vi "4461 Autophase.vi"(8 "error in (no error)":errorcluster, 9 "Boolean":bool, 10 "Results":T1 {"Results (Dictionary)"."value" format="%#_6p"}, 11 "Instrument.DAQ in":refnum<class "Instrument.DAQ.lvclass">) -> (0 "error out":errorcluster, 3 "Instrument.DAQ out":refnum<class "Instrument.DAQ.lvclass">)   [LabVIEW 2019, in "Instrument.DAQ.lvclass"]
uses:
  Instrument.DAQ.lvclass
  Typedefs/Results--Cluster.ctl
  Instrument.Lockin/Typedefs/Results Type--Enum.ctl
  Instrument.DAQ.lvclass/Instrument.DAQ.ctl
  <vilib>/addons/control/pid/pid.llb/PID (DBL Array).vi
  Instrument.Lockin/Instrument.Lockin.lvclass
  <vilib>/addons/control/pid/NI_PID_pid.lvlib
  <vilib>/addons/control/pid/pid.llb/PID Control Input Filter (DBL).vi
panel:
  out "output":dbl[](array[numeric]) format="%.2f"
  in  "D":dbl=0.019999999999999997 format="%.3f"
  in  "I":dbl=0.6 format="%.3f"
  in  "P":dbl=0.5 format="%.2f"
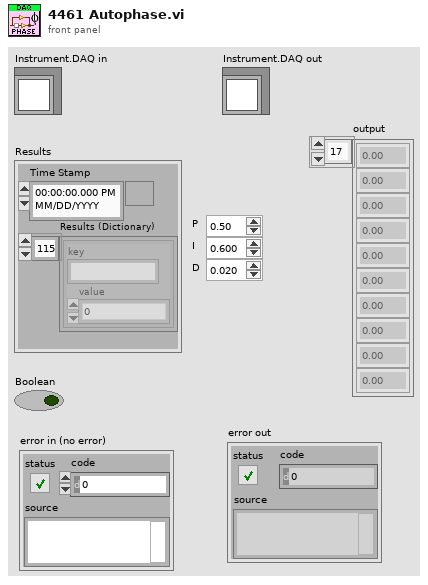
[diagram p1: front panel]
types:
  T1 = typedef "Instrument.DAQ.lvclass/Results--Cluster.ctl" = cluster{"Time Stamp":timestamp, "Results (Dictionary)":cluster{"key":string, "value":dbl}[]}
  T2 = cluster{"proportional gain (Kc)":dbl, "integral time (Ti, min)":dbl, "derivative time (Td, min)":dbl}
  T3 = typedef "Instrument.Lockin.lvclass/Results Type--Enum.ctl" = enum16{"X", "Y", "R", "Theta", "Mean"}
  T4 = typedef "Instrument.DAQ.lvclass/AO.Channel--Cluster--Array.ctl" = T5[]
  T5 = typedef "Instrument.DAQ.lvclass/AO.Channel--Cluster.ctl" = cluster{"Enable?":bool, "Channel":i32, "Amplitude":dbl, "Offset":dbl, "Frequency":dbl, "Phase":dbl, "Function":T6, "Sweeping?":bool}
  T6 = typedef "Instrument.DAQ.lvclass/AO.Channel.Function--Enum.ctl" = enum16{"Sine", "Triangle", "Square"}
  T7 = cluster{"proportional gain (Kc)":dbl, "integral time (Ti, min)":dbl, "derivative time (Td, min)":dbl}[]
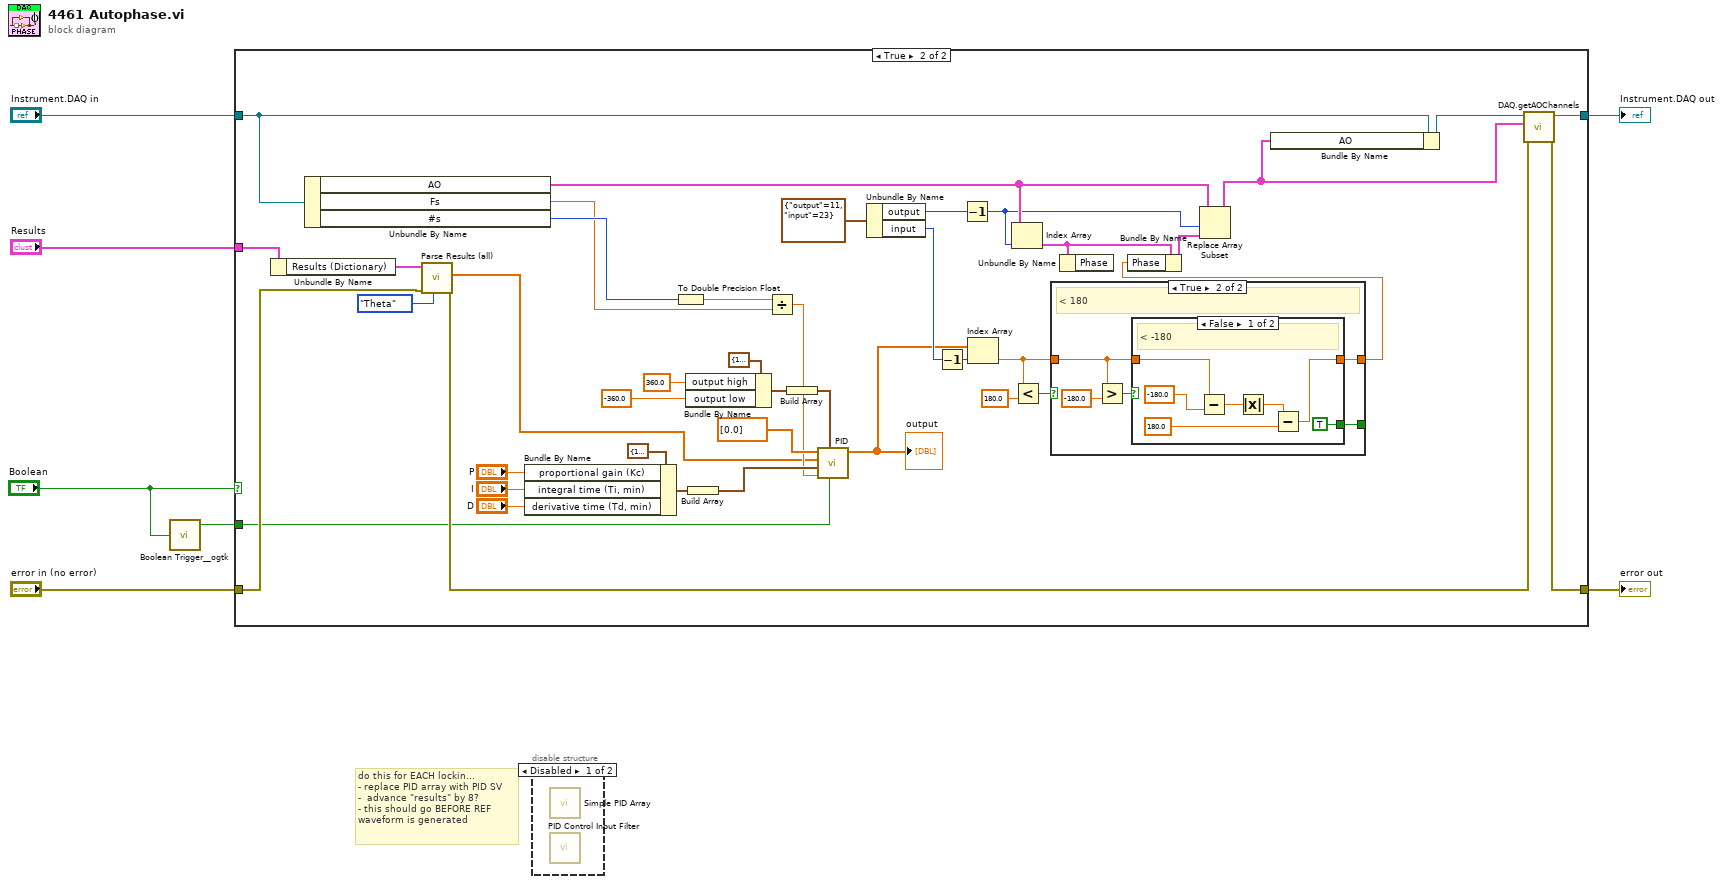
[diagram p0: block diagram]
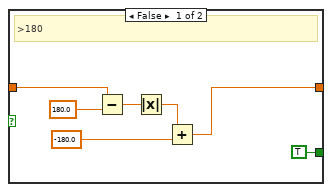
[diagram p3: hidden frame]
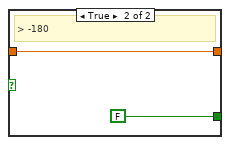
[diagram p4: hidden frame]
diagram:
  # "do this for EACH lockin...\n- replace PID array with PID SV\n-  advance \"results\" by 8?\n- this should go BEFORE REF\nwaveform is generated"
  n1 = call <userlib>:"Boolean Trigger__ogtk.vi"("Boolean Input"="Boolean") -> ("Rising Edge"=w1:bool)  [unwired: 1 in, 1 out]
  n2 = case shown="True" "Boolean" {
    tunnel: "Instrument.DAQ in" -> [w9 w50]
    tunnel: "Results" -> [_ w49]
    tunnel: "error in (no error)" -> [w8 w48]
    tunnel: [w9 w47] -> w4
    tunnel: [w8 w11] -> w3
    tunnel: w1 -> [_ w10]
    frame False {
    }
    frame True {
      n3 = Unbundle By Name(w49) -> ("Results (Dictionary)"=w46:cluster{"key":string, "value":dbl}[])
      n4 = Unbundle By Name(w50) -> ("AO"=w30:T4, "Fs"=w20:dbl, "#s"=w21:i32)
      n5 = call "Parse Results (all).vi"("Type"=Results_Type--Enum."Theta", "error in (no error)"=w48, "Results (Dictionary)"=w46) -> ("error out"=w43:errorcluster, "Data"=w12:dbl[])  [unwired: 5 in, 2 out]
      n6 = Bundle By Name(cluster=T2 {"proportional gain (Kc)"=1.0, "integral time (Ti, min)"=0.01, "derivative time (Td, min)"=0.0} ("PID gains"), "proportional gain (Kc)"="P", "integral time (Ti, min)"="I", "derivative time (Td, min)"="D") -> (w36:T2)
      n7 = To Double Precision Float(number=w21) -> (double precision float=w13:dbl)
      n8 = Bundle By Name(cluster=cluster{"output high":dbl, "output low":dbl} {"output high"=100.0, "output low"=-100.0} ("output range"), "output high"=360.0, "output low"=-360.0) -> (w37:cluster{"output high":dbl, "output low":dbl})
      n9 = Build Array(w36) -> (w32:T7)
      n10 = Divide(x=w13, y=w20) -> (x/y=w19:dbl)
      n11 = Build Array(w37) -> (w28:cluster{"output high":dbl, "output low":dbl}[])
      n12 = call-poly <vilib>:"PID.vi"("reinitialize? (F)"=w10, "output range"=w28, "dt (s)"=w19, "PID gains"=w32, "process variable"=w12, "setpoint"=dbl[] [0.0]) -> ("output"=w18:dbl[])  [unwired: 4 in, 1 out]
      "output" <- w18
      n13 = Unbundle By Name(cluster{"output":i32, "input":i32} {"output"=11, "input"=23}) -> ("output"=w26:i32, "input"=w25:i32)
      n14 = Decrement(x=w25) -> (x-1=w24:i32)
      n15 = Decrement(x=w26) -> (x-1=w23:i32)
      n16 = Index Array(array=w18, index=w24) -> (element=w15:dbl)
      n17 = Index Array(array=w30, index=w23) -> (element=w31:T5)
      n18 = Less?(x=w15, y=180.0) -> (x < y?=w16:bool)
      n19 = case shown="True" w16 {
        tunnel: w15 -> [w53 w59]
        tunnel: [w52 w60] -> w14
        tunnel: [TRUE w58] -> _
        frame False {
          # ">180"
          n20 = Subtract(x=w53, y=180.0) -> (x-y=w56:dbl)
          n21 = Absolute Value(x=w56) -> (abs(x)=w55:dbl)
          n22 = Add(x=w55, y=-180.0) -> (x+y=w52:dbl)
        }
        frame True {
          # "< 180"
          n23 = Greater?(x=w59, y=-180.0) -> (0:w62:bool)
          n24 = case shown="False" w62 {
            tunnel: [w64 w71] -> w60
            tunnel: w59 -> [w65 w71]
            tunnel: [TRUE FALSE] -> w58
            frame False {
              # "< -180"
              n25 = Subtract(x=w65, y=-180.0) -> (x-y=w68:dbl)
              n26 = Absolute Value(x=w68) -> (abs(x)=w67:dbl)
              n27 = Subtract(x=w67, y=180.0) -> (x-y=w64:dbl)
            }
            frame True {
              # "> -180"
            }
          }
        }
      }
      n28 = Unbundle By Name(w31) -> ()  [unwired: 1 out]
      n29 = Bundle By Name(cluster=w31, "Phase"=w14) -> (w29:T5)
      n30 = Replace Array Subset(array=w30, new element=w29, index=w23) -> (w22:T4)
      n31 = Bundle By Name(cluster=w50, "AO"=w22) -> (w44:refnum<class "Instrument.DAQ.lvclass">)
      n32 = call "DAQ.getAOChannels.vi"("error in (no error)"=w43, "Channels: AO"=w22, "Instrument.DAQ"=w44) -> ("error out"=w11:errorcluster, "Instrument.DAQ out"=w47:refnum<class "Instrument.DAQ.lvclass">)  [unwired: 7 in]
    }
  }
  "Instrument.DAQ out" <- w4
  "error out" <- w3
  n33 = disable-structure shown="Disabled" {
    frame Disabled {
      n34 = call "Simple PID Array.vi"() -> ()  [unwired: 11 in, 1 out]
      n35 = call-poly <vilib>:"PID Control Input Filter.vi"() -> ()  [unwired: 5 in, 1 out]
    }
    frame Enabled {
    }
  }
